vi "Array of String_Memory Block.vi"(6 "Group Indices":i32[](array[numeric]), 8 "Data In":cluster{"String Array":string[]}[](array[cluster]), 9 "Value":cluster{"String Array":string[]}, 10 "Index":i32, 11 "Method":T1=enum."Read") -> (0 "Group Data":cluster{"String Array":string[]}[](array[cluster]), 3 "Value Out":cluster{"String Array":string[]}, 5 "Array Size/Current Index":i32)   [LabVIEW 2020]
doc: "This functional global variable stores all of the actual data for the tags in the CVT. All IO goes through this VI."
uses:
  Type Defs/Memory Commands.ctl
  Current Value Table(Rebuild).lvlib
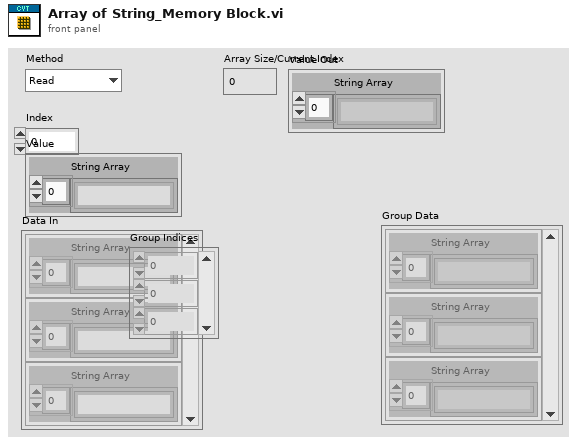
[diagram p1: front panel]
types:
  T1 = typedef "Current Value Table(Rebuild).lvlib/Memory Commands.ctl" = enum16{"Init", "Add Data", "Read", "Read Group", "Read All", "Write", "Write Group", "Get Size"}
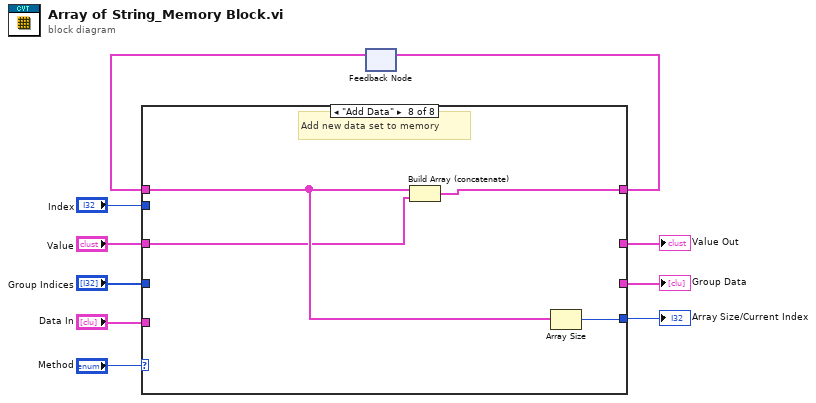
[diagram p0: block diagram]
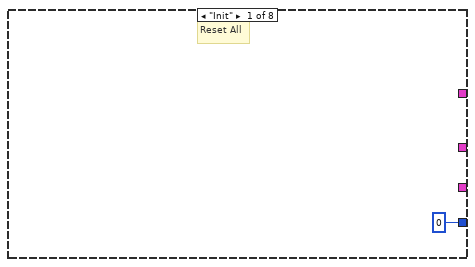
[diagram p2: hidden frame]
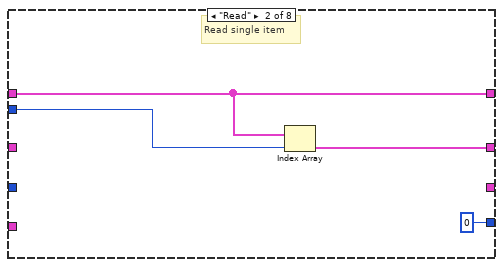
[diagram p3: hidden frame]
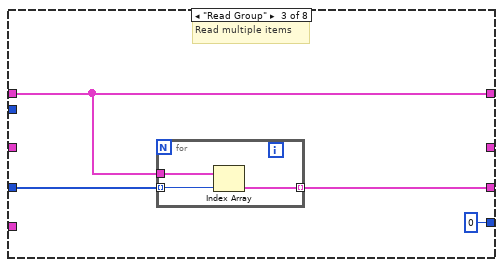
[diagram p4: hidden frame]
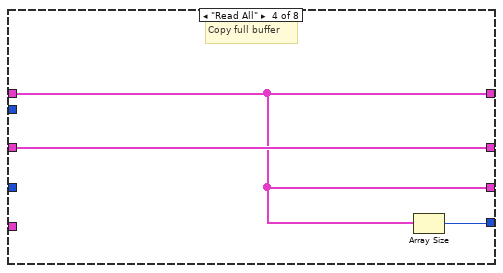
[diagram p5: hidden frame]
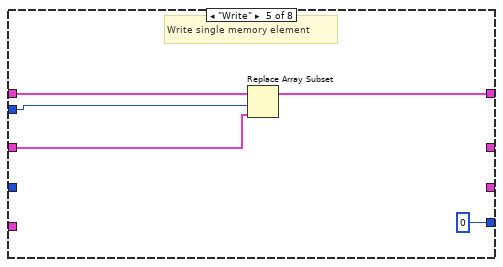
[diagram p6: hidden frame]
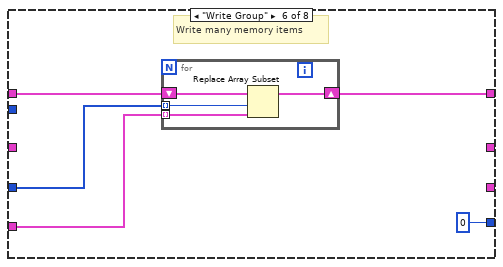
[diagram p7: hidden frame]
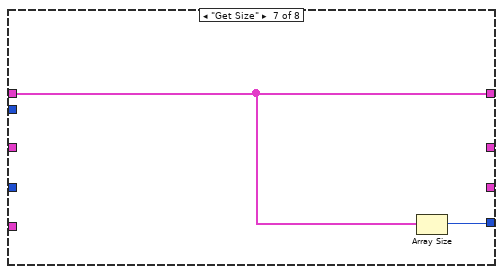
[diagram p8: hidden frame]
diagram:
  n1 = feedback #1() -> (w1:cluster{"String Array":string[]}[])  [unwired: 1 in]
  n2 = case shown="\"Add Data\"" "Method" {
    tunnel: [_ w12 w16 w23 w28 w34 w41 w45] -> w2
    tunnel: w1 -> [_ w12 w16 w23 w30 w35 w41 w43]
    tunnel: "Value" -> [_ _ _ w25 w26 _ _ w42]
    tunnel: [_ w14 _ w25 _ _ _ _] -> w3
    tunnel: "Index" -> [_ w13 _ _ w29 _ _ _]
    tunnel: "Data In" -> [_ _ _ _ _ w31 _ _]
    tunnel: [0 ("Index") 0 ("Index") 0 ("Index") w24 0 ("Index") 0 ("Index") w40 w44] -> w7
    tunnel: "Group Indices" -> [_ _ w19 _ _ w33 _ _]
    tunnel: [_ _ w18 w23 _ _ _ _] -> w5
    frame "Init" {
      # "Reset All"
    }
    frame "Read" {
      # "Read single item"
      n3 = Index Array(array=w12, index=w13) -> (element=w14:cluster{"String Array":string[]})
    }
    frame "Read Group" {
      # "Read multiple items"
      n4 = for {
        tunnel: w19 -> [w21] mode=indexing
        tunnel: [w22] -> w18 mode=indexing
        tunnel: w16 -> [w20]
        n5 = Index Array(array=w20, index=w21) -> (element=w22:cluster{"String Array":string[]})
      }
    }
    frame "Read All" {
      # "Copy full buffer"
      n6 = Array Size(array=w23) -> (size(s)=w24:i32)
    }
    frame "Write" {
      # "Write single memory element"
      n7 = Replace Array Subset(array=w30, new element=w26, index=w29) -> (w28:cluster{"String Array":string[]}[])
    }
    frame "Write Group" {
      # "Write many memory items"
      n8 = for {
        shift-right: [w38] -> w34
        shift-left: w35 -> [w39]
        tunnel: w33 -> [w37] mode=indexing
        tunnel: w31 -> [w36] mode=indexing
        n9 = Replace Array Subset(array=w39, new element=w36, index=w37) -> (w38:cluster{"String Array":string[]}[])
      }
    }
    frame "Get Size" {
      n10 = Array Size(array=w41) -> (size(s)=w40:i32)
    }
    frame "Add Data" {
      # "Add new data set to memory"
      n11 = Build Array (concatenate)(w43, w42) -> (w45:cluster{"String Array":string[]}[])
      n12 = Array Size(array=w43) -> (size(s)=w44:i32)
    }
  }
  "Array Size/Current Index" <- w7
  "Group Data" <- w5
  "Value Out" <- w3
  n13 = feedback-in #1(w2) -> ()
